vi "断电保存全局.vi"() -> ()   [LabVIEW 2016]
panel:
  in  "url":string="http://47.92.120.37:3020/api/v1/wuz_hours"
  in  "station_id":string="123456"
  in  "time":string="2021-05-08 14:02:02"
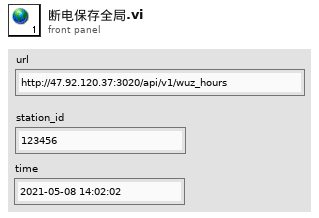
[diagram p1: front panel]
diagram:
